vi "Day08-2.vi"() -> ()   [LabVIEW 2021]
uses:
  9a3c5581-57cc-4c88-af3e-ab8df778c4ed.vi
  4bec7fdc-367e-4fec-9492-2eb2bf652b8f.vi
  c8f50ca9-b5f3-4055-8225-49cd2d035d61.vi
  <vilib>/Comparison/Less/Less Functor/Less Functor.lvclass
panel:
  out "sum":i32
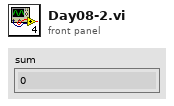
[diagram p1: front panel]
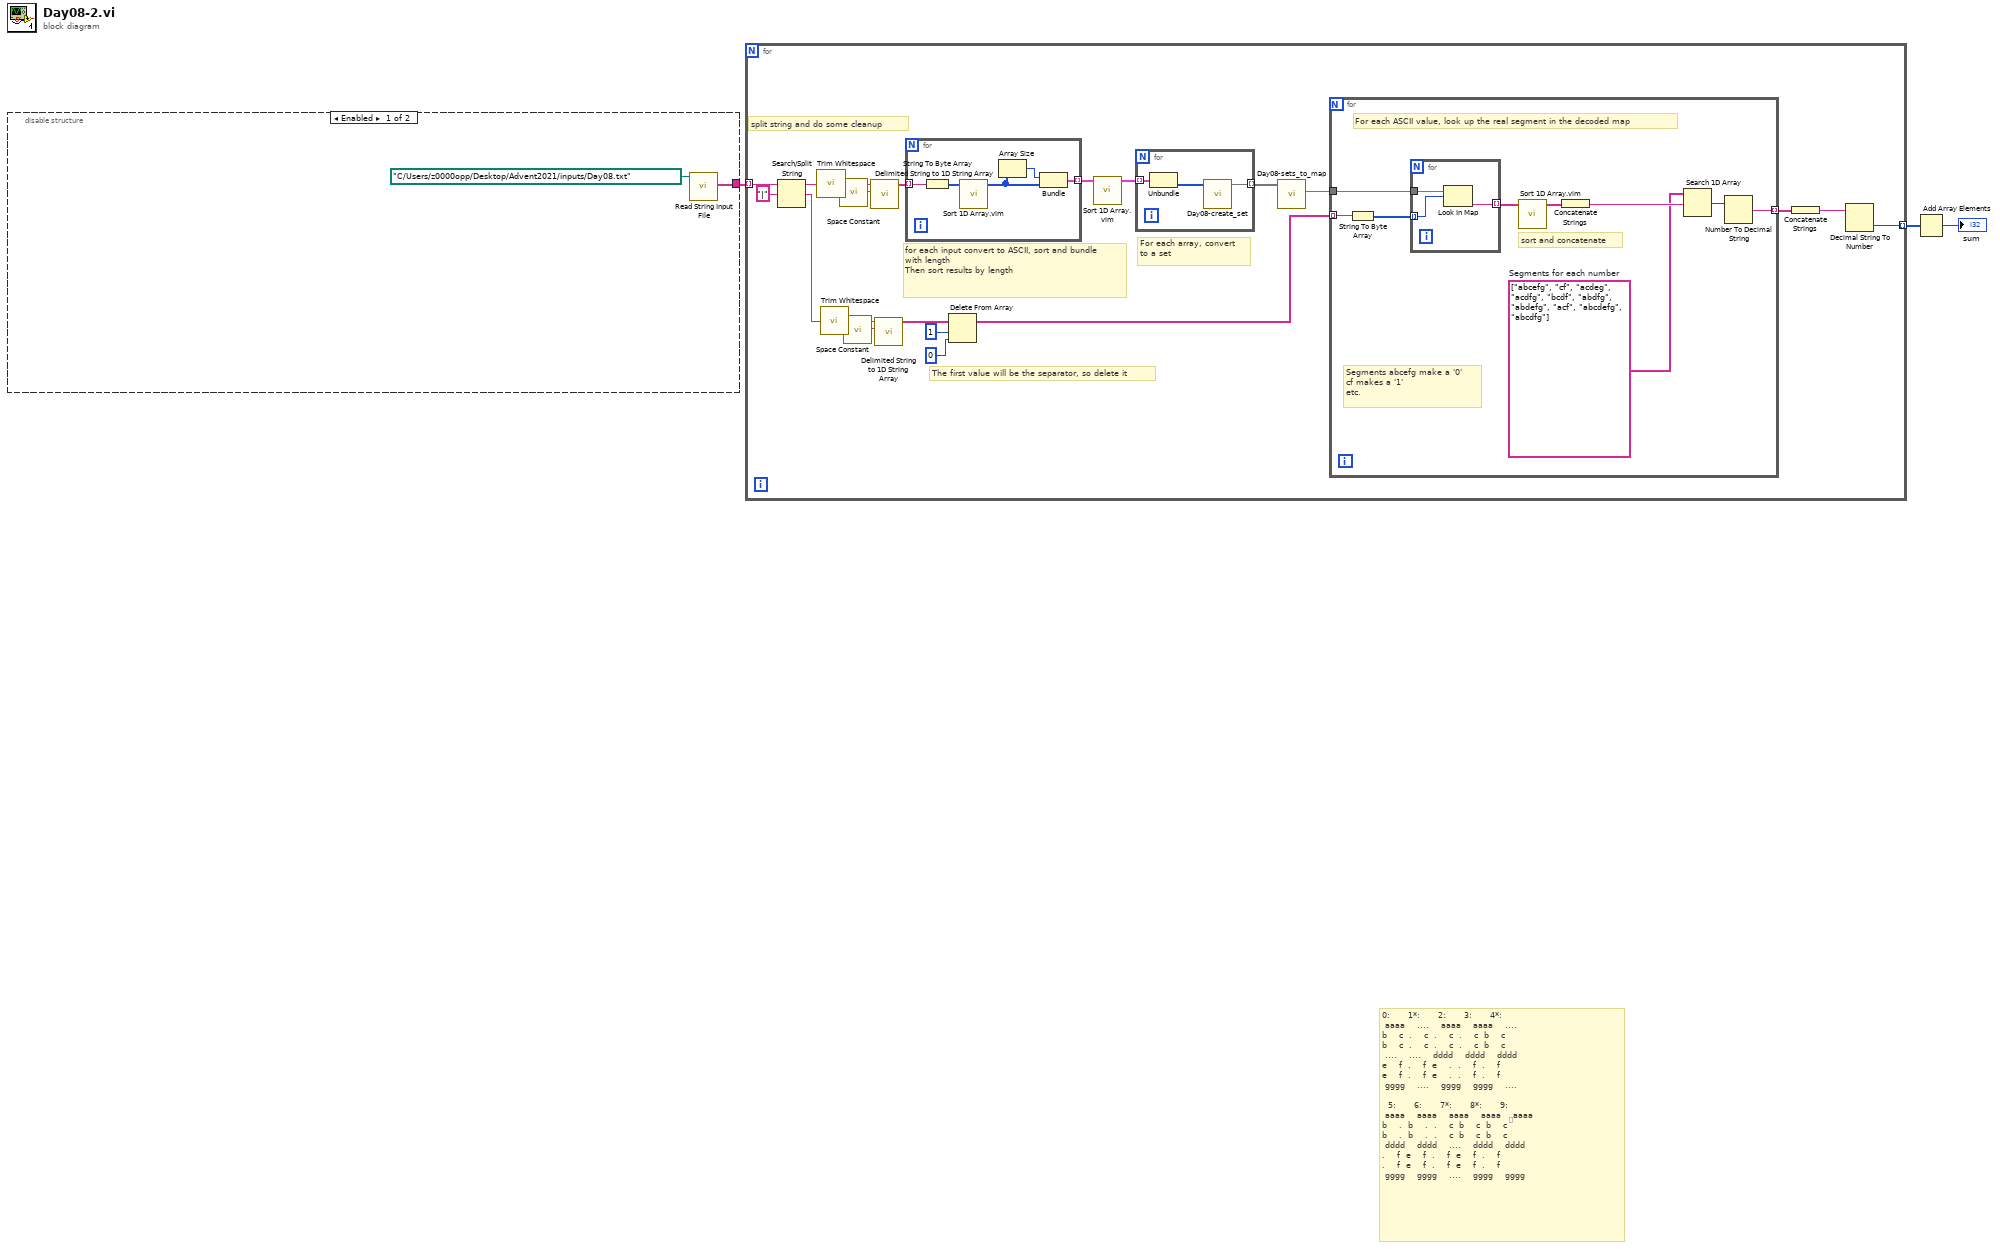
[diagram p0: block diagram]
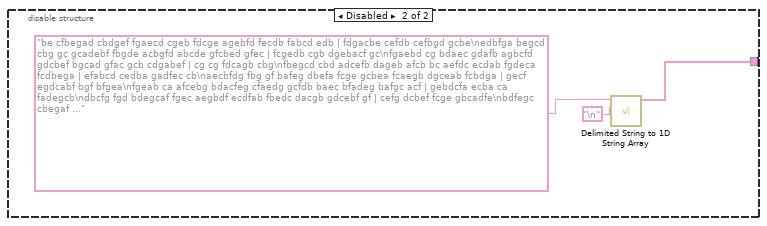
[diagram p2: hidden frame]
diagram:
  # "0:      1*:      2:      3:      4*:\n aaaa    ....    aaaa    aaaa    ....\nb    c  .    c  .    c  .    c  b    c\nb    c  .    c  .    c  .    c  b    c\n ....    ....    dddd    dddd    dddd\ne    f  .    f  e    .  .    f  .    f\ne    f  .    f  e    .  .    f  .    f\n gggg    ....    gggg    gggg    ....\n\n  5:      6:      7*:      8*:      9:\n aaaa    aaaa    aaaa    aaaa    aaaa\nb    .  b    .  .    c  b    c  b    c\nb    .  b    .  .    c  b    c  b    c\n dddd    dddd    ....    dddd    dddd\n.    f  e    f  .    f  e    f  .    f\n.    f  e    f  .    f  e    f  .    f\n gggg    gggg    ....    gggg    gggg"
  n1 = disable-structure shown="Enabled" {
    disable-tunnel: [w4 w6] -> w3
    frame Enabled {
      n2 = call "Read String Input File.vi"("file path (dialog if empty)"=path "C:/Users/z0000opp/Desktop/Advent2021/inputs/Day08.txt") -> ("input values"=w4:string[])  [unwired: 10 in]
    }
    frame Disabled {
      n3 = call <vilib>:"Delimited String to 1D String Array.vi"("delimiter"="\n", "delimited string"="be cfbegad cbdgef fgaecd cgeb fdcge agebfd fecdb fabcd edb | fdgacbe cefdb cefbgd gcbe\nedbfga begcd cbg gc gcadebf fbgde acbgfd abcde gfcbed gfec | fcgedb cgb dgebacf gc\nfgaebd cg bdaec gdafb agbcfd gdcbef bgcad gfac gcb cdgabef | cg cg fdcagb cbg\nfbegcd cbd adcefb dageb afcb bc aefdc ecdab fgdeca fcdbega | efabcd cedba gadfec cb\naecbfdg fbg gf bafeg dbefa fcge gcbea fcaegb dgceab fcbdga | gecf egdcabf bgf bfgea\nfgeab ca afcebg bdacfeg cfaedg gcfdb baec bfadeg bafgc acf | gebdcfa ecba ca fadegcb\ndbcfg fgd bdegcaf fgec aegbdf ecdfab fbedc dacgb gdcebf gf | cefg dcbef fcge gbcadfe\nbdfegc cbegaf gecbf dfcage bdacg ed bedf ced adcbefg gebcd | ed bcgafe cdgba cbgef\negadfb cdbfeg cegd fecab cgb gbdefca cg fgcdab egfdb bfceg | gbdfcae bgc cg cgb\ngcafb gcf dcaebfg ecagb gf abcdeg gaef cafbge fdbac fegbdc | fgae cfgab fg bagce") -> ("string array"=w6:string[])  [unwired: 9 in]
    }
  }
  n4 = for {
    tunnel: w3 -> [w25] mode=indexing
    tunnel: [w12] -> w2 mode=indexing
    # "The first value will be the separator, so delete it"
    # "For each array, convert\nto a set"
    # "for each input convert to ASCII, sort and bundle with length\nThen sort results by length"
    # "split string and do some cleanup"
    n5 = Search/Split String(string=w25, search string/char (-)="|") -> (substring before match=w24:string, match + rest of string=w18:string)  [unwired: 1 in, 1 out]
    n6 = call <vilib>:"Trim Whitespace.vi"("string"=w24) -> ("trimmed string"=w27:string)  [unwired: 1 in]
    n7 = call <vilib>:"Trim Whitespace.vi"("string"=w18) -> ("trimmed string"=w23:string)  [unwired: 1 in]
    n8 = call <vilib>:"Space Constant.vi"() -> ("String"=w26:string)
    n9 = call <vilib>:"Space Constant.vi"() -> ("String"=w22:string)
    n10 = call <vilib>:"Delimited String to 1D String Array.vi"("delimiter"=w26, "delimited string"=w27) -> ("string array"=w17:string[])  [unwired: 9 in]
    n11 = call <vilib>:"Delimited String to 1D String Array.vi"("delimiter"=w22, "delimited string"=w23) -> ("string array"=w21:string[])  [unwired: 9 in]
    n12 = for {
      tunnel: w17 -> [w45] mode=indexing
      tunnel: [w46] -> w16 mode=indexing
      n13 = String To Byte Array(string=w45) -> (unsigned byte array=w44:u8[])
      n14 = call "Sort 1D Array.vim"("unsorted array"=w44) -> ("sorted array"=w48:u8[])  [unwired: 10 in]
      n15 = Array Size(array=w48) -> (size(s)=w47:i32)
      n16 = Bundle(w47, "sorted array"=w48) -> (w46:cluster{i32, "sorted array":u8[]})  [unwired: 1 in]
    }
    n17 = Delete From Array(array=w21, length=1, index=0) -> (array with subset deleted=w13:string[])  [unwired: 1 out]
    n18 = call "Sort 1D Array.vim"("unsorted array"=w16) -> ("sorted array"=w15:cluster{i32, "sorted array":u8[]}[])  [unwired: 10 in]
    n19 = for {
      tunnel: w15 -> [w43] mode=indexing
      tunnel: [w41] -> w14 mode=indexing
      n20 = Unbundle(w43) -> ("sorted array"=w42:u8[])  [unwired: 1 out]
      n21 = call "Day08-create_set.vi"("sorted array"=w42) -> ("Set"=w41:set{u8})  [unwired: 10 in]
    }
    n22 = call "Day08-sets_to_map.vi"("Array of sets"=w14) -> ("map"=w11:map{u8, string})  [unwired: 10 in]
    n23 = for {
      tunnel: w13 -> [w37] mode=indexing
      tunnel: w11 -> [w35]
      tunnel: [w32] -> w10 mode=indexing
      w29 = string[] ["abcefg", "cf", "acdeg", "acdfg", "bcdf", "abdfg", "abdefg", "acf", "abcdefg", "abcdfg"]  # Segments for each number
      # "Segments abcefg make a '0'\ncf makes a '1'\netc."
      # "sort and concatenate"
      # "For each ASCII value, look up the real segment in the decoded map"
      n24 = String To Byte Array(string=w37) -> (unsigned byte array=w36:u8[])
      n25 = for {
        tunnel: w36 -> [w39] mode=indexing
        tunnel: w35 -> [w40]
        tunnel: [w38] -> w34 mode=indexing
        n26 = Look In Map(map=w40, key=w39) -> (value=w38:string)  [unwired: 1 in, 1 out]
      }
      n27 = call "Sort 1D Array.vim"("unsorted array"=w34) -> ("sorted array"=w31:string[])  [unwired: 10 in]
      n28 = Concatenate Strings(w31) -> (w30:string)
      n29 = Search 1D Array(1D array=w29, element=w30) -> (index of element=w33:i32)  [unwired: 1 in]
      n30 = Number To Decimal String(number=w33) -> (decimal integer string=w32:string)  [unwired: 1 in]
    }
    n31 = Concatenate Strings(w10) -> (w9:string)
    n32 = Decimal String To Number(string=w9) -> (number=w12:i32)  [unwired: 2 in, 1 out]
  }
  n33 = Add Array Elements(numeric array=w2) -> (sum=→"sum":i32)
